vi "Configure Display Trace.vi"(6 "Measurement Name (MY_MEAS)":string="MY_MEAS", 7 "Mode (0: Create)":u16(ring) items=["Create", "Delete"], 8 "Error In (no error)":errorcluster, 9 "Display Trace (1)":i32=1, 10 "Display Window (1)":i32=1, 11 "VISA Resource Name":refnum<visa-resource-name>) -> (0 "Error Out":errorcluster, 3 "VISA Resource Name Out":refnum<visa-resource-name>)   [LabVIEW 2018, in "Agilent PNA Series.lvlib"]
doc: "This VI creates or deletes a display trace in the selected window. \n\nNote: If the window doesn't exist (in Create mode), then VI will create it. If the trace already exists, the current measurement assigned to that trace would be replaced."
uses:
  Agilent PNA Series.lvlib
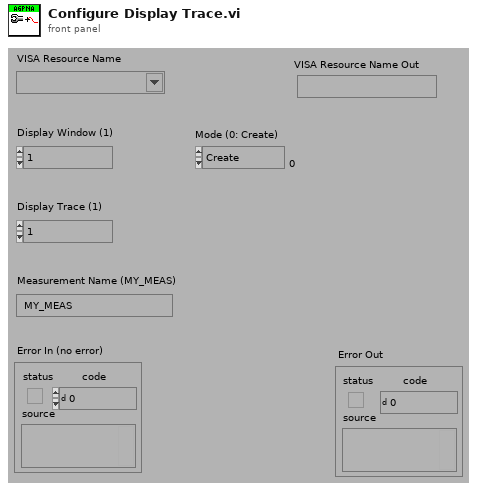
[diagram p1: front panel]
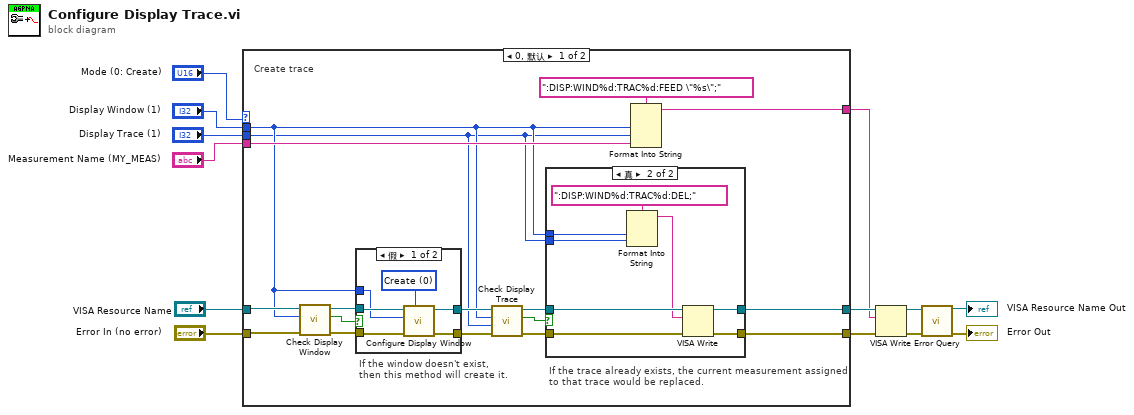
[diagram p0: block diagram]
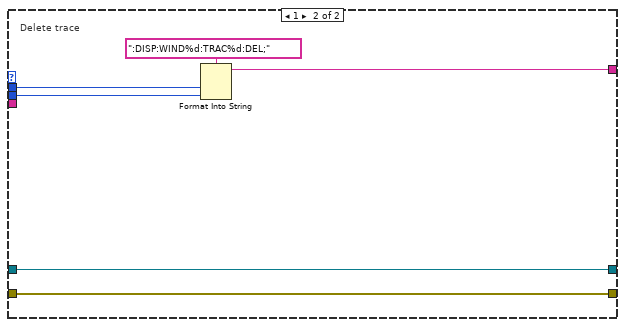
[diagram p4: hidden frame]
diagram:
  n1 = case shown="0, 默认" "Mode (0: Create)" {
    tunnel: "Measurement Name (MY_MEAS)" -> [w16 _]
    tunnel: "Display Trace (1)" -> [w14 w53]
    tunnel: "Display Window (1)" -> [w15 w52]
    tunnel: [w29 w51] -> w5
    tunnel: "VISA Resource Name" -> [w27 w50]
    tunnel: [w19 w50] -> w8
    tunnel: "Error In (no error)" -> [w28 w49]
    tunnel: [w20 w49] -> w6
    frame 0, Default {
      # "If the trace already exists, the current measurement assigned \nto that trace would be replaced."
      # "If the window doesn't exist,\nthen this method will create it."
      # "Create trace"
      n2 = call "Check Display Window.vi"("Error In (no error)"=w28, "Display Window (1)"=w15, "VISA Resource Name"=w27) -> ("Error Out"=w25:errorcluster, "Display Window Check"=w24:bool, "VISA Resource Name Out"=w26:refnum<visa-resource-name>)  [unwired: 5 in, 1 out]
      n3 = case shown="假" w24 {
        tunnel: w26 -> [w46 w48]
        tunnel: [w45 w48] -> w23
        tunnel: w25 -> [w44 w47]
        tunnel: [w43 w47] -> w22
        tunnel: w15 -> [w42 _]
        frame False {
          w41 = u16 0 items=["Create", "Delete"] ("Mode (0: Create)")
          n4 = call "Configure Display Window.vi"("Mode (0: Create)"=w41, "Error In (no error)"=w44, "Display Window (1)"=w42, "VISA Resource Name"=w46) -> ("Error Out"=w43:errorcluster, "VISA Resource Name Out"=w45:refnum<visa-resource-name>)  [unwired: 6 in]
        }
        frame True {
        }
      }
      n5 = call "Check Display Trace.vi"("Error In (no error)"=w22, "Display Trace (1)"=w14, "Display Window (1)"=w15, "VISA Resource Name"=w23) -> ("Error Out"=w21:errorcluster, "Display Trace Check"=w17:bool, "VISA Resource Name Out"=w18:refnum<visa-resource-name>)  [unwired: 4 in, 1 out]
      n6 = case shown="真" w17 {
        tunnel: w21 -> [w32 w34]
        tunnel: [w32 w35] -> w20
        tunnel: [w31 w36] -> w19
        tunnel: w18 -> [w31 w37]
        tunnel: w15 -> [_ w39]
        tunnel: w14 -> [_ w38]
        frame False {
        }
        frame True {
          n7 = Format Into String(format string=":DISP:WIND%d:TRAC%d:DEL;", w39, w38) -> (resulting string=w33:string)  [unwired: 2 in, 1 out]
          n8 = VISA Write(VISA resource name=w37, write buffer=w33, error in (no error)=w34) -> (VISA resource name out=w36:refnum<visa-resource-name>, error out=w35:errorcluster)  [unwired: 1 out]
        }
      }
      n9 = Format Into String(format string=":DISP:WIND%d:TRAC%d:FEED \"%s\";", w15, w14, w16) -> (resulting string=w29:string)  [unwired: 2 in, 1 out]
    }
    frame 1 {
      # "Delete trace"
      n10 = Format Into String(format string=":DISP:WIND%d:TRAC%d:DEL;", w52, w53) -> (resulting string=w51:string)  [unwired: 2 in, 1 out]
    }
  }
  n11 = VISA Write(VISA resource name=w8, write buffer=w5, error in (no error)=w6) -> (VISA resource name out=w4:refnum<visa-resource-name>, error out=w3:errorcluster)  [unwired: 1 out]
  n12 = call "Error Query.vi"("VISA Resource Name"=w4, "error in (no error)"=w3) -> ("VISA Resource Name Out"=→"VISA Resource Name Out":refnum<visa-resource-name>, "error out"=→"Error Out":errorcluster)  [unwired: 10 in, 2 out]
